vi "HB Latency.vi"(10 "HB":string) -> (2 "HB Latency ms":u32, 3 "HB Rx":u32)   [LabVIEW 2018]
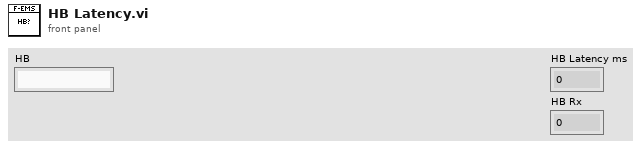
[diagram p1: front panel]
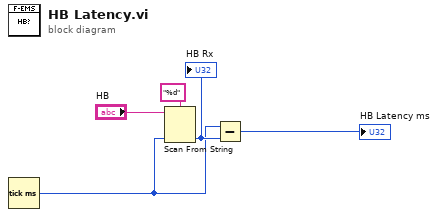
[diagram p0: block diagram]
diagram:
  n1 = Tick Count (ms)() -> (millisecond timer value=w2:u32)
  n2 = Scan From String(format string="%d", input string="HB", default 1=w2) -> (output 1=w3:u32)  [unwired: 2 in, 3 out]
  "HB Rx" <- w3
  n3 = Subtract(x=w2, y=w3) -> (x-y=→"HB Latency ms":u32)
